vi "DSP_send_command.vi"(0 "Value":dbl, 1 "CMD selection":T1(ring), 2 "GPIB address":string="0:12") -> ()   [LabVIEW 2013]
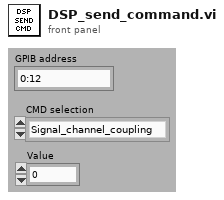
[diagram p1: front panel]
types:
  T1 = enum16{"Signal_channel_coupling", "Signal_channel_input_mode", "SC_FET_BIPOLAR", "SC_LineFilter", "Auto_ac_gain", "AC_gain", "Sensitivity", "Auto_sensitivity", "Auto_phase", "Auto_sensitivity_phase", "Time_constant", "Reference_channel_source", "Oscillator_amplitude", "Oscilllator_frequency"}
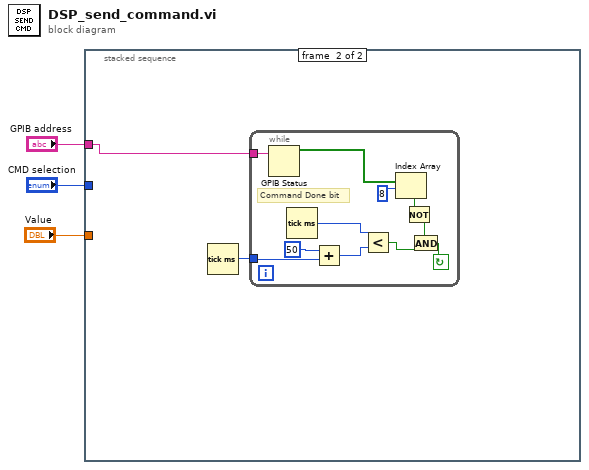
[diagram p0: block diagram]
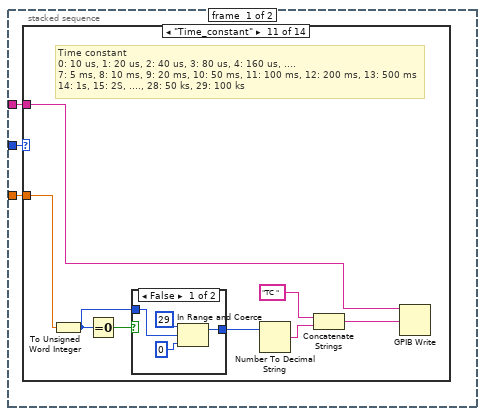
[diagram p2: hidden frame]
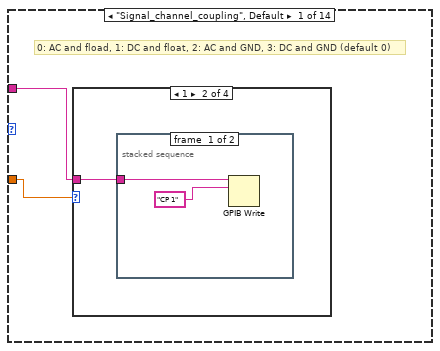
[diagram p3: hidden frame]
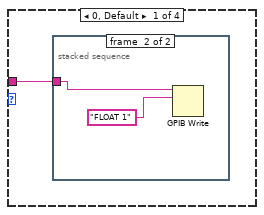
[diagram p4: hidden frame]
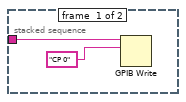
[diagram p5: hidden frame]
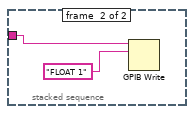
[diagram p6: hidden frame]
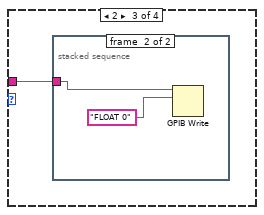
[diagram p7: hidden frame]
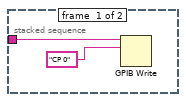
[diagram p8: hidden frame]
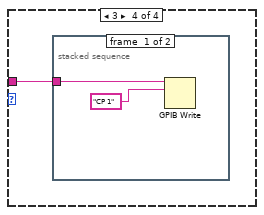
[diagram p9: hidden frame]
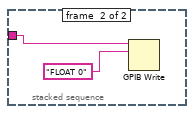
[diagram p10: hidden frame]
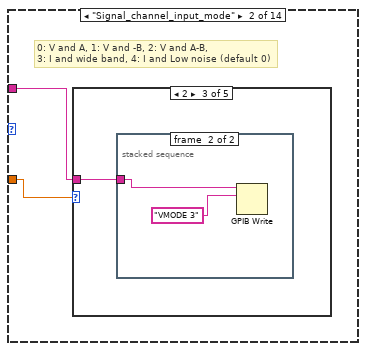
[diagram p11: hidden frame]
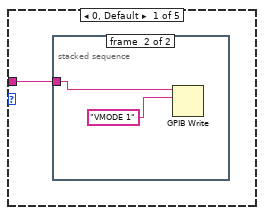
[diagram p12: hidden frame]
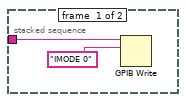
[diagram p13: hidden frame]
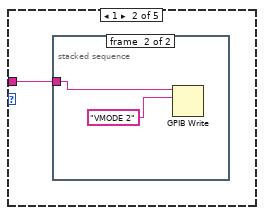
[diagram p14: hidden frame]
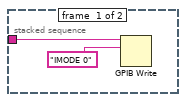
[diagram p15: hidden frame]
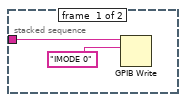
[diagram p16: hidden frame]
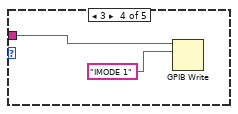
[diagram p17: hidden frame]
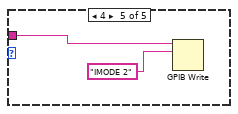
[diagram p18: hidden frame]
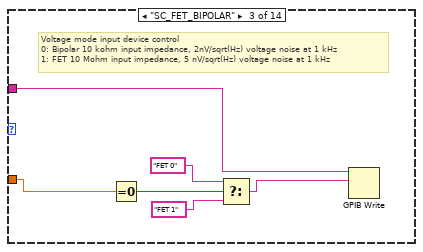
[diagram p19: hidden frame]
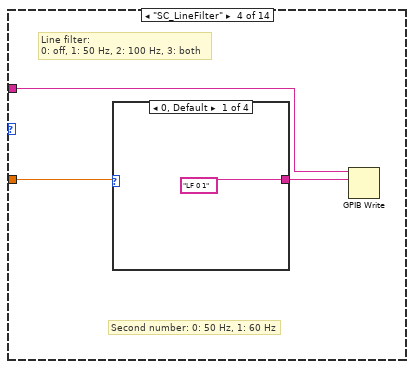
[diagram p20: hidden frame]
diagram:
  n1 = stacked-sequence {
    tunnel: "CMD selection" -> [w6 _]
    tunnel: "Value" -> [w5 _]
    tunnel: "GPIB address" -> [w4 w151]
    frame #0 {
      n2 = case shown="\"Time_constant\"" w6 {
        tunnel: w5 -> [w8 w30 w50 w58 w63 w70 w85 w98 w103 w108 w111 w124 w134 w144]
        tunnel: w4 -> [w7 w29 w51 w56 w64 w71 w90 w96 w101 w106 w112 w125 w138 w148]
        frame "Signal_channel_coupling", Default {
          # "0: AC and fload, 1: DC and float, 2: AC and GND, 3: DC and GND (default 0)"
          n3 = case shown="1" w8 {
            tunnel: w7 -> [w9 w14 w19 w24]
            frame 0, Default {
              n4 = stacked-sequence {
                tunnel: w9 -> [w10 w12]
                frame #0 {
                  n5 = GPIB Write(0:w10, 1:"CP 0") -> ()  [unwired: 3 in, 2 out]
                }
                frame #1 {
                  n6 = GPIB Write(0:w12, 1:"FLOAT 1") -> ()  [unwired: 3 in, 2 out]
                }
              }
            }
            frame 1 {
              n7 = stacked-sequence {
                tunnel: w14 -> [w15 w17]
                frame #0 {
                  n8 = GPIB Write(0:w15, 1:"CP 1") -> ()  [unwired: 3 in, 2 out]
                }
                frame #1 {
                  n9 = GPIB Write(0:w17, 1:"FLOAT 1") -> ()  [unwired: 3 in, 2 out]
                }
              }
            }
            frame 2 {
              n10 = stacked-sequence {
                tunnel: w19 -> [w20 w22]
                frame #0 {
                  n11 = GPIB Write(0:w20, 1:"CP 0") -> ()  [unwired: 3 in, 2 out]
                }
                frame #1 {
                  n12 = GPIB Write(0:w22, 1:"FLOAT 0") -> ()  [unwired: 3 in, 2 out]
                }
              }
            }
            frame 3 {
              n13 = stacked-sequence {
                tunnel: w24 -> [w25 w27]
                frame #0 {
                  n14 = GPIB Write(0:w25, 1:"CP 1") -> ()  [unwired: 3 in, 2 out]
                }
                frame #1 {
                  n15 = GPIB Write(0:w27, 1:"FLOAT 0") -> ()  [unwired: 3 in, 2 out]
                }
              }
            }
          }
        }
        frame "Signal_channel_input_mode" {
          # "0: V and A, 1: V and -B, 2: V and A-B,\n3: I and wide band, 4: I and Low noise (default 0)"
          n16 = case shown="2" w30 {
            tunnel: w29 -> [w31 w36 w41 w47 w49]
            frame 0, Default {
              n17 = stacked-sequence {
                tunnel: w31 -> [w32 w34]
                frame #0 {
                  n18 = GPIB Write(0:w32, 1:"IMODE 0") -> ()  [unwired: 3 in, 2 out]
                }
                frame #1 {
                  n19 = GPIB Write(0:w34, 1:"VMODE 1") -> ()  [unwired: 3 in, 2 out]
                }
              }
            }
            frame 1 {
              n20 = stacked-sequence {
                tunnel: w36 -> [w37 w39]
                frame #0 {
                  n21 = GPIB Write(0:w37, 1:"IMODE 0") -> ()  [unwired: 3 in, 2 out]
                }
                frame #1 {
                  n22 = GPIB Write(0:w39, 1:"VMODE 2") -> ()  [unwired: 3 in, 2 out]
                }
              }
            }
            frame 2 {
              n23 = stacked-sequence {
                tunnel: w41 -> [w42 w44]
                frame #0 {
                  n24 = GPIB Write(0:w42, 1:"IMODE 0") -> ()  [unwired: 3 in, 2 out]
                }
                frame #1 {
                  n25 = GPIB Write(0:w44, 1:"VMODE 3") -> ()  [unwired: 3 in, 2 out]
                }
              }
            }
            frame 3 {
              n26 = GPIB Write(0:w47, 1:"IMODE 1") -> ()  [unwired: 3 in, 2 out]
            }
            frame 4 {
              n27 = GPIB Write(0:w49, 1:"IMODE 2") -> ()  [unwired: 3 in, 2 out]
            }
          }
        }
        frame "SC_FET_BIPOLAR" {
          # "Voltage mode input device control\n0: Bipolar 10 kohm input impedance, 2nV/sqrt(Hz) voltage noise at 1 kHz\n1: FET 10 Mohm input impedance, 5 nV/sqrt(Hz) voltage noise at 1 kHz"
          n28 = Equal To 0?(x=w50) -> (x = 0?=w55:bool)
          n29 = Select(t="FET 0", s=w55, f="FET 1") -> (s? t:f=w52:string)
          n30 = GPIB Write(0:w51, 1:w52) -> ()  [unwired: 3 in, 2 out]
        }
        frame "SC_LineFilter" {
          # "Second number: 0: 50 Hz, 1: 60 Hz"
          # "Line filter:\n0: off, 1: 50 Hz, 2: 100 Hz, 3: both"
          n31 = case shown="0, Default" w58 {
            tunnel: ["LF 0 1" "LF 1 1" "LF 2 1" "LF 3 1"] -> w57
            frame 0, Default {
            }
            frame 1 {
            }
            frame 2 {
            }
            frame 3 {
            }
          }
          n32 = GPIB Write(0:w56, 1:w57) -> ()  [unwired: 3 in, 2 out]
        }
        frame "Auto_ac_gain" {
          # "Auto ac gain\n0: off, 1: on"
          n33 = Equal To 0?(x=w63) -> (x = 0?=w65:bool)
          n34 = Select(t="AUTOMATIC 0", s=w65, f="AUTOMATIC 1") -> (s? t:f=w68:string)
          n35 = GPIB Write(0:w64, 1:w68) -> ()  [unwired: 3 in, 2 out]
        }
        frame "AC_gain" {
          # "AC gain\n0 ~ 9 --> 0 dB ~ 90 dB in 10 dB step"
          n36 = To Unsigned Byte Integer(number=w70) -> (unsigned 8bit integer=w69:u8)
          n37 = case shown="9" w69 {
            tunnel: ["ACGAIN 0" "ACGAIN 1" "ACGAIN 2" "ACGAIN 3" "ACGAIN 4" "ACGAIN 5" "ACGAIN 6" "ACGAIN 7" "ACGAIN 8" "ACGAIN 9"] -> w72
            frame 0, Default {
            }
            frame 1 {
            }
            frame 2 {
            }
            frame 3 {
            }
            frame 4 {
            }
            frame 5 {
            }
            frame 6 {
            }
            frame 7 {
            }
            frame 8 {
            }
            frame 9 {
            }
          }
          n38 = GPIB Write(0:w71, 1:w72) -> ()  [unwired: 3 in, 2 out]
        }
        frame "Sensitivity" {
          # "Sensitivity\n1: 2nV, 2: 5 nV, 3: 10 nV\n4: 20 nV, 5: 50 nV, 6: 100 nV\n...\n25: 200 mV, 26: 500 mV, 27: 1 V\n\nCalculation:\n10^(floor(N/3)-1)*[2 or 5 or 10, corresponding to N mod 3] nV"
          n39 = To Unsigned Word Integer(number=w85) -> (unsigned 16bit integer=w83:u16)
          n40 = Equal To 0?(x=w83) -> (x = 0?=w86:bool)
          n41 = case shown="False" w86 {
            tunnel: w83 -> [w93 _]
            tunnel: [w94 27] -> w84
            frame False {
              n42 = In Range and Coerce(upper limit=27, x=w93, lower limit=1) -> (coerced(x)=w94:i32)  [unwired: 1 out]
            }
            frame True {
            }
          }
          n43 = Number To Decimal String(number=w84) -> (decimal integer string=w89:string)  [unwired: 1 in]
          n44 = Concatenate Strings("SEN ", w89) -> (w87:string)
          n45 = GPIB Write(0:w90, 1:w87) -> ()  [unwired: 3 in, 2 out]
        }
        frame "Auto_sensitivity" {
          # "Auto sensitivice\n0: nothing, else: auto sensitivity"
          n46 = Not Equal To 0?(x=w98) -> (x != 0?=w97:bool)
          n47 = case shown="True" w97 {
            tunnel: w96 -> [_ w99]
            frame False {
            }
            frame True {
              n48 = GPIB Write(0:w99, 1:"AS") -> ()  [unwired: 3 in, 2 out]
            }
          }
        }
        frame "Auto_phase" {
          # "Auto phase\n0: nothing, else: auto sensitivity"
          n49 = Not Equal To 0?(x=w103) -> (x != 0?=w102:bool)
          n50 = case shown="True" w102 {
            tunnel: w101 -> [_ w104]
            frame False {
            }
            frame True {
              n51 = GPIB Write(0:w104, 1:"AQN") -> ()  [unwired: 3 in, 2 out]
            }
          }
        }
        frame "Auto_sensitivity_phase" {
          # "Auto phase\n0: nothing, else: auto sensitivity"
          n52 = Not Equal To 0?(x=w108) -> (x != 0?=w107:bool)
          n53 = case shown="True" w107 {
            tunnel: w106 -> [_ w109]
            frame False {
            }
            frame True {
              n54 = GPIB Write(0:w109, 1:"ASM") -> ()  [unwired: 3 in, 2 out]
            }
          }
        }
        frame "Time_constant" {
          # "Time constant\n0: 10 us, 1: 20 us, 2: 40 us, 3: 80 us, 4: 160 us, ....\n7: 5 ms, 8: 10 ms, 9: 20 ms, 10: 50 ms, 11: 100 ms, 12: 200 ms, 13: 500 ms\n14: 1s, 15: 2S, ...., 28: 50 ks, 29: 100 ks"
          n55 = To Unsigned Word Integer(number=w111) -> (unsigned 16bit integer=w118:u16)
          n56 = Equal To 0?(x=w118) -> (x = 0?=w116:bool)
          n57 = case shown="False" w116 {
            tunnel: w118 -> [w121 _]
            tunnel: [w122 27] -> w117
            frame False {
              n58 = In Range and Coerce(upper limit=29, x=w121, lower limit=0) -> (coerced(x)=w122:i32)  [unwired: 1 out]
            }
            frame True {
            }
          }
          n59 = Number To Decimal String(number=w117) -> (decimal integer string=w113:string)  [unwired: 1 in]
          n60 = Concatenate Strings("TC ", w113) -> (w115:string)
          n61 = GPIB Write(0:w112, 1:w115) -> ()  [unwired: 3 in, 2 out]
        }
        frame "Reference_channel_source" {
          # "Reference channel\n0: internal, 1: External logic (external rear panel TTL input)\n2: External (external front panel input)"
          n62 = To Unsigned Byte Integer(number=w124) -> (unsigned 8bit integer=w127:u8)
          n63 = case shown="0, Default" w127 {
            tunnel: ["IE 0" "IE 1" "IE 2"] -> w126
            frame 0, Default {
            }
            frame 1 {
            }
            frame 2 {
            }
          }
          n64 = GPIB Write(0:w125, 1:w126) -> ()  [unwired: 3 in, 2 out]
        }
        frame "Oscillator_amplitude" {
          # "Osillcator amplitude (V rms)"
          n65 = In Range and Coerce(upper limit=5.00000001, x=w134, lower limit=0.0) -> (coerced(x)=w133:dbl)  [unwired: 1 out]
          n66 = Multiply(x=w133, y=1000000) -> (x*y=w136:dbl)
          n67 = Number To Decimal String(number=w136) -> (decimal integer string=w135:string)  [unwired: 1 in]
          n68 = Concatenate Strings("OA ", w135) -> (w139:string)
          n69 = GPIB Write(0:w138, 1:w139) -> ()  [unwired: 3 in, 2 out]
        }
        frame "Oscilllator_frequency" {
          # "Osillcator frequency (Hz)"
          n70 = In Range and Coerce(upper limit=250000.0001, x=w144, lower limit=0.0) -> (coerced(x)=w143:dbl)  [unwired: 1 out]
          n71 = Multiply(x=w143, y=1000) -> (x*y=w146:dbl)
          n72 = Number To Decimal String(number=w146) -> (decimal integer string=w145:string)  [unwired: 1 in]
          n73 = Concatenate Strings("OF ", w145) -> (w149:string)
          n74 = GPIB Write(0:w148, 1:w149) -> ()  [unwired: 3 in, 2 out]
        }
      }
    }
    frame #1 {
      n75 = Tick Count (ms)() -> (millisecond timer value=w152:u32)
      n76 = while {
        tunnel: w152 -> [w157]
        tunnel: w151 -> [w156]
        stop <- w159 continue-if-true
        # "Command Done bit"
        n77 = GPIB Status(0:w156) -> (2:w155:bool[])  [unwired: 1 in, 3 out]
        n78 = Tick Count (ms)() -> (millisecond timer value=w162:u32)
        n79 = Add(x=u32 50, y=w157) -> (x+y=w161:u32)
        n80 = Less?(x=w162, y=w161) -> (x < y?=w158:bool)
        n81 = Index Array(array=w155, index=8) -> (element=w154:bool)
        n82 = Not(x=w154) -> (.not. x?=w153:bool)
        n83 = And(x=w153, y=w158) -> (x .and. y?=w159:bool)
      }
    }
  }
